vi "Parse Branch Return.vi"(11 "standard output":string="  SMO\n* develop\n  master\n") -> (2 "branches":string[](array[string]), 3 "active branch":string)   [LabVIEW 2019, in "Git.lvclass"]
uses:
  Git.lvclass
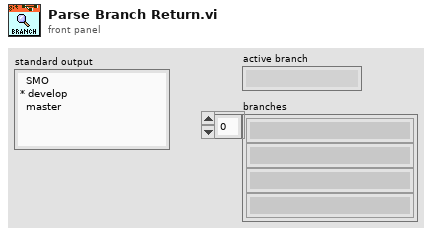
[diagram p1: front panel]
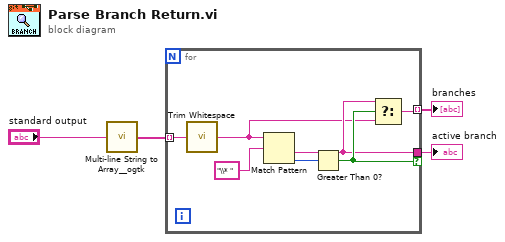
[diagram p0: block diagram]
diagram:
  n1 = call <userlib>:"Multi-line String to Array__ogtk.vi"("string"="standard output") -> ("lines"=w1:string[])
  n2 = for {
    tunnel: [w9] -> w4 if=w11
    tunnel: w1 -> [w8] mode=indexing
    tunnel: [w10] -> w3 mode=indexing
    n3 = call <vilib>:"Trim Whitespace.vi"("string"=w8) -> ("trimmed string"=w5:string)  [unwired: 1 in]
    n4 = Match Pattern(string=w5, regular expression="\\* ") -> (after substring=w9:string, offset past match=w6:i32)  [unwired: 1 in, 2 out]
    n5 = Greater Than 0?(x=w6) -> (x > 0?=w11:bool)
    n6 = Select(t=w9, s=w11, f=w5) -> (s? t:f=w10:string)
  }
  "active branch" <- w4
  "branches" <- w3
